vi "SW_Gen_Draw_numbers_and_highllights_DAQmx.vi"(5 "Regions to mark selected":u16[](array[numeric]), 6 "Colors cluster":T2, 7 "Regions to mark set":u16[](array[numeric]), 8 "Input cluster of parameters":T3={"Cage diameter, mm"=8, "Starting angle MIDFIELD"=0, "Starting angle BORDER"=4, "Radius, mm CENTER"=0, "Radius, mm MIDFIELD"=60, "N segments MIDFIELD"=1, "N segments BORDER"=30, "R-gap, mm"=180.0, "Bridge swap"=FALSE, "Bridge H. offset"=0.0, "Bridge V. offset"=0.0, "Twisted neck"=FALSE, "Alt. magn. orientation"=FALSE, "Sensor board size"=enum."Small"} {"Cage diameter, mm" scale=0.0..340.0}, 9 "Image geometrical and scaling parameters":T4, 10 "Bounding rectangles":T5, 11 "Experiment Diagram":T1(plugin-control)) -> (3 "Experiment Diagram out":T1(plugin-control))   [LabVIEW 2018, in "Tracker.lvlib"]
uses:
  Tracker.lvlib
  Controls/CTL_Bounding_Rectangle_of_Segments.ctl
  Controls/CTL_Image_Geometrical_and_scaling_parameters.ctl
  Controls/CTL_Segmented_plot_parameters.ctl
panel:
  in  "Bigger bubble radius":i32=15
  in  "Bubble radius":i16=11
  in  "Font size":i16=18
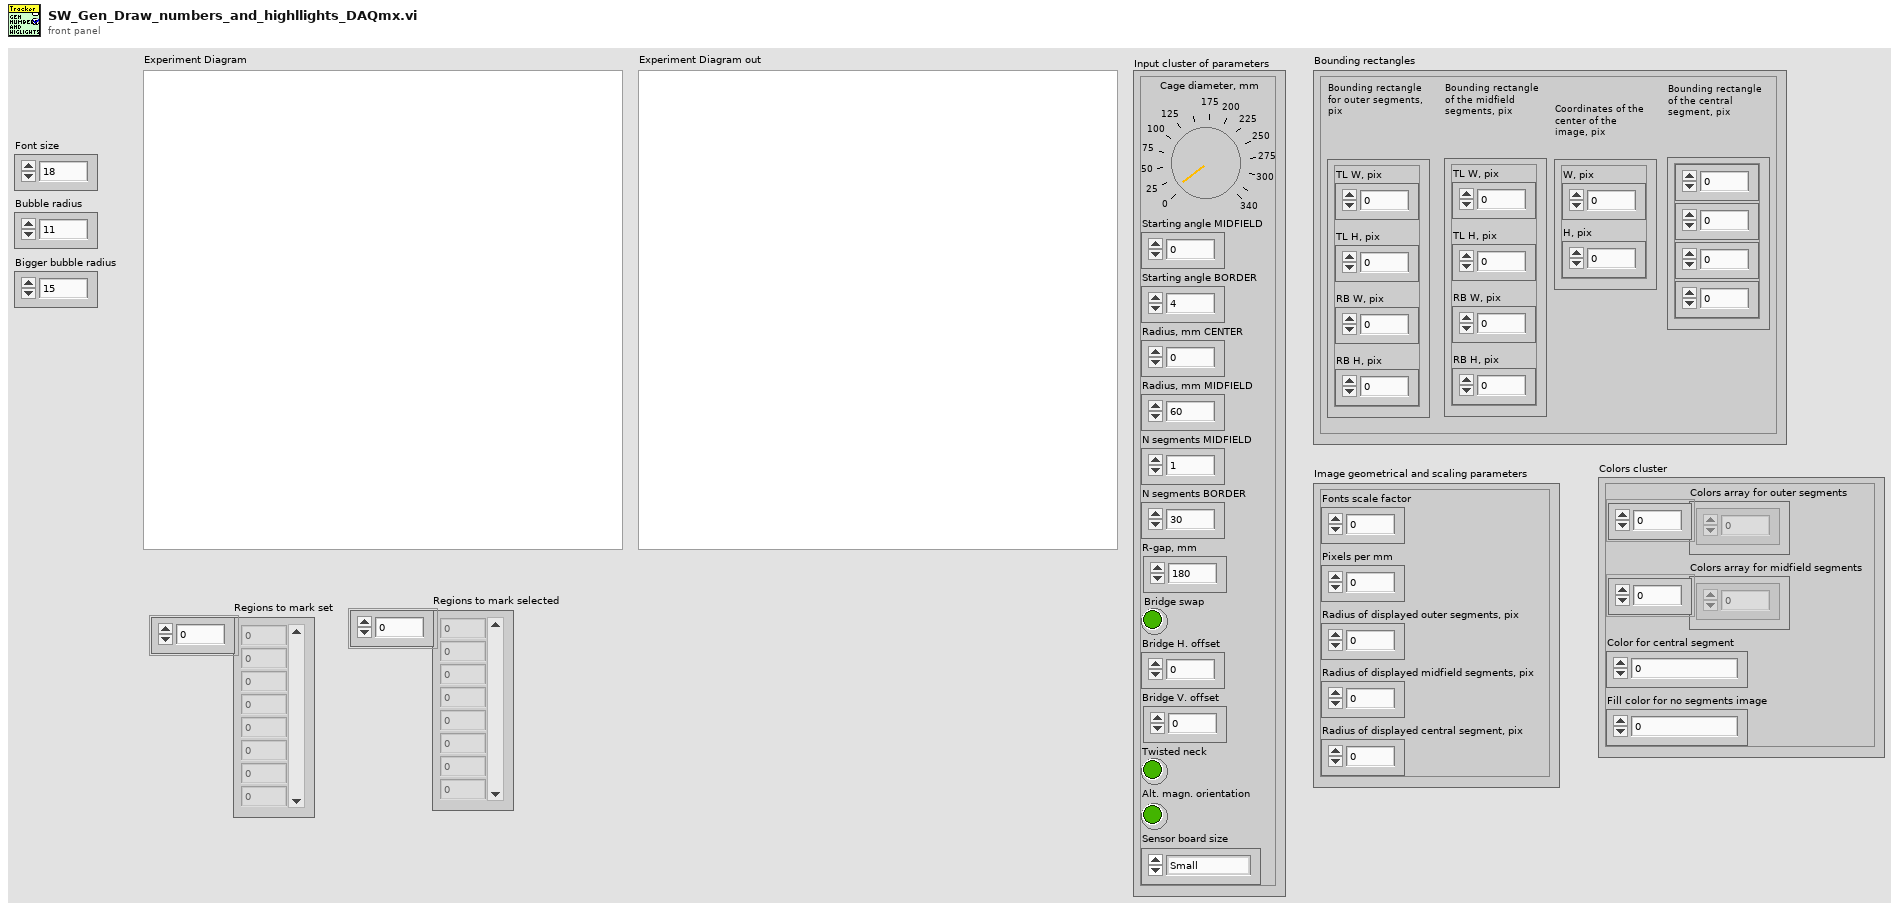
[diagram p1: front panel]
types:
  T1 = typedef "IMAQ Image.ctl" = refnum<image>
  T2 = cluster{"Colors array for outer segments":u32[], "Colors array for midfield segments":u32[], "Color for central segment":u32, "Fill color for no segments image":u32}
  T3 = typedef "Tracker.lvlib/CTL_Segmented_plot_parameters.ctl" = cluster{"Cage diameter, mm":u16, "Starting angle MIDFIELD":i16, "Starting angle BORDER":i16, "Radius, mm CENTER":u16, "Radius, mm MIDFIELD":u16, "N segments MIDFIELD":u8, "N segments BORDER":u8, "R-gap, mm":sgl, "Bridge swap":bool, "Bridge H. offset":sgl, "Bridge V. offset":sgl, "Twisted neck":bool, "Alt. magn. orientation":bool, "Sensor board size":enum16{"Small", "Large"}}
  T4 = typedef "Tracker.lvlib/CTL_Image_Geometrical_and_scaling_parameters.ctl" = cluster{"Fonts scale factor":dbl, "Pixels per mm":dbl, "Radius of displayed outer segments, pix":dbl, "Radius of displayed midfield segments, pix":dbl, "Radius of displayed central segment, pix":dbl}
  T5 = typedef "Tracker.lvlib/CTL_Bounding_Rectangle_of_Segments.ctl" = cluster{"Bounding rectangle for outer segments, pix":cluster{"TL W, pix":i32, "TL H, pix":i32, "RB W, pix":i32, "RB H, pix":i32}, "Bounding rectangle of the midfield segments, pix":cluster{"TL W, pix":i32, "TL H, pix":i32, "RB W, pix":i32, "RB H, pix":i32}, "Coordinates of the center of the image, pix":cluster{"W, pix":i32, "H, pix":i32}, "Bounding rectangle of the central segment, pix":cluster{"Numeric Control":i32, "Numeric Control":i32, "Numeric Control":i32, "Numeric Control":i32}}
  T6 = cluster{"TL W, pix":i32, "TL H, pix":i32, "RB W, pix":i32, "RB H, pix":i32}
  T7 = cluster{"Desired Font (Application)":enum16{"User-specified Font", "Application Font", "System Font", "Dialog Font"}, "[User-specified Font]":cluster{"Font Name":string, "Size":i16, "Strikeout?":bool, "Italic?":bool, "Underline?":bool, "Outline?":bool, "Shadow?":bool, "Bold?":bool, "Rotation Angle":dbl}, "Horizontal Alignment":i16, "Vertical Alignment":i16}
  T8 = cluster{"Top":i32, "Left":i32, "Bottom":i32, "Right":i32}
  T9 = enum16{"User-specified Font", "Application Font", "System Font", "Dialog Font"}
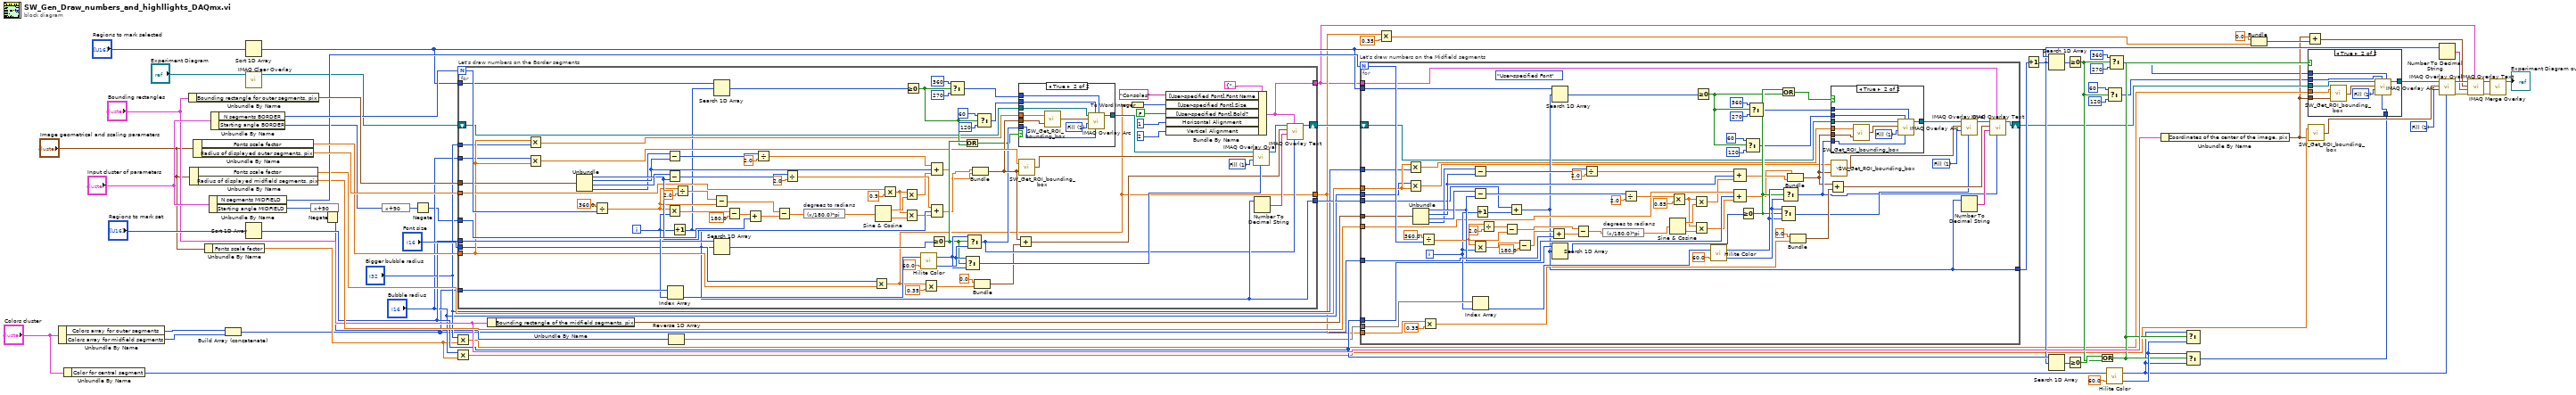
[diagram p0: block diagram]
diagram:
  w27 = u32 1 items=["Frame", "Fill"] ("Drawing Mode (Frame)")
  n1 = Unbundle By Name("Colors cluster") -> ("Colors array for outer segments"=w38:u32[], "Colors array for midfield segments"=w37:u32[])
  n2 = Unbundle By Name("Colors cluster") -> ("Color for central segment"=w52:u32)
  n3 = Unbundle By Name("Bounding rectangles") -> ("Bounding rectangle for outer segments, pix"=w70:T6)
  n4 = Unbundle By Name("Image geometrical and scaling parameters") -> ("Fonts scale factor"=w63:dbl, "Radius of displayed midfield segments, pix"=w62:dbl)
  n5 = Unbundle By Name("Image geometrical and scaling parameters") -> ("Fonts scale factor"=w68:dbl, "Radius of displayed outer segments, pix"=w69:dbl)
  n6 = Unbundle By Name("Image geometrical and scaling parameters") -> ("Fonts scale factor"=w39:dbl)
  n7 = Unbundle By Name("Input cluster of parameters") -> ("N segments MIDFIELD"=w65:u8, "Starting angle MIDFIELD"=w7:i16)
  n8 = Unbundle By Name("Input cluster of parameters") -> ("N segments BORDER"=w67:u8, "Starting angle BORDER"=w8:i16)
  n9 = Build Array (concatenate)(w38, w37) -> (w36:u32[])
  n10 = Sort 1D Array(array="Regions to mark selected") -> (sorted array=w47:u16[])
  n11 = call "IMAQ Clear Overlay"("Image"="Experiment Diagram") -> ("Image Out"=w33:T1)  [unwired: 9 in, 1 out]
  n12 = Sort 1D Array(array="Regions to mark set") -> (sorted array=w51:u16[])
  n13 = expression code="x+90"(w7) -> (w5:i16)
  n14 = Negate(x=w5) -> (-x=w3:i16)
  n15 = expression code="x+90"(w8) -> (w6:i16)
  n16 = Negate(x=w6) -> (-x=w4:i16)
  n17 = Multiply(x="Bigger bubble radius", y=w39) -> (x*y=w30:dbl)
  n18 = Multiply(x="Bubble radius", y=w39) -> (x*y=w19:dbl)
  n19 = for "Let's draw numbers on the Border segments" {
    N: w67 -> [w152]
    tunnel: w4 -> [w153]
    tunnel: w70 -> [w147]
    tunnel: w36 -> [w126]
    tunnel: w69 -> [w123]
    tunnel: w51 -> [w120]
    tunnel: w68 -> [w113]
    tunnel: w47 -> [w112]
    tunnel: "Font size" -> [w106]
    tunnel: "Bubble radius" -> [w105]
    tunnel: "Bigger bubble radius" -> [w104]
    tunnel: [w98] -> w60
    shift-right: [w94] -> w32
    shift-left: w33 -> [w102]
    tunnel: [w79] -> w15
    tunnel: [w78] -> w13
    i -> [w125]
    w97 = u32 1 items=["Frame", "Fill"] ("Drawing Mode (Frame)")
    n20 = Multiply(x=w113, y=w104) -> (x*y=w103:dbl)
    n21 = Multiply(x=w105, y=w113) -> (x*y=w99:dbl)
    n22 = Unbundle(w147) -> ("TL W, pix"=w141:i32, "TL H, pix"=w134:i32, "RB W, pix"=w146:i32, "RB H, pix"=w133:i32)
    n23 = Divide(x=360.0, y=w152) -> (x/y=w127:dbl)
    n24 = Subtract(x=w133, y=w134) -> (x-y=w136:i32)
    n25 = Subtract(x=w146, y=w141) -> (x-y=w144:i32)
    n26 = Multiply(x=w127, y=w125) -> (x*y=w131:dbl)
    n27 = Index Array(array=w126, index=w125) -> (element=w117:u32)
    n28 = Increment(x=w125) -> (x+1=w98:i32)
    n29 = Divide(x=w127, y=2.0) -> (x/y=w129:dbl)
    n30 = Search 1D Array(1D array=w112, element=w98) -> (index of element=w111:i32)  [unwired: 1 in]
    n31 = Subtract(x=w129, y=w127) -> (x-y=w128:dbl)
    n32 = Search 1D Array(1D array=w120, element=w98) -> (index of element=w119:i32)  [unwired: 1 in]
    n33 = Subtract(x=w131, y=180.0) -> (x-y=w132:dbl)
    n34 = Add(x=w132, y=w153) -> (x+y=w150:dbl)
    n35 = Divide(x=w136, y=2.0) -> (x/y=w138:dbl)
    n36 = Subtract(x=w128, y=w150) -> (x-y=w149:dbl)
    n37 = Divide(x=w144, y=2.0) -> (x/y=w142:dbl)
    n38 = expression code="(x/180.0)*pi" "degrees to radians"(w149) -> (w148:dbl)
    n39 = Multiply(x=w106, y=w113) -> (x*y=w79:dbl)
    n40 = Sine & Cosine(0:w148) -> (1:w135:dbl, 2:w145:dbl)
    n41 = Multiply(x=w123, y=0.9) -> (x*y=w122:dbl)
    n42 = Multiply(x=w122, y=w135) -> (x*y=w139:dbl)
    n43 = Multiply(x=w122, y=w145) -> (x*y=w140:dbl)
    n44 = Greater Or Equal To 0?(x=w111) -> (x >= 0?=w108:bool)
    n45 = call <vilib>:"Hilite Color.vi"("Percentage(30)"=60.0, "Color In"=w117) -> ("Shadow"=w116:u32, "Hilite"=w115:u32)
    n46 = Multiply(x=w79, y=0.35) -> (x*y=w84:dbl)
    n47 = Greater Or Equal To 0?(x=w119) -> (x >= 0?=w114:bool)
    n48 = Compound Arithmetic op=ADD(w138, w134, w139) -> (w74:dbl)
    n49 = Compound Arithmetic op=ADD(w142, w141, w140) -> (w75:dbl)
    n50 = Select(t=i16 360, s=w108, f=i16 270 ("arc size(360)")) -> (s? t:f=w76:i16)
    n51 = Or(x=w114, y=w108) -> (x .or. y?=w80:bool)
    n52 = Select(t=w116, s=w114, f=w115) -> (s? t:f=w96:u32)
    n53 = Select(t=w115, s=w114, f=w116) -> (s? t:f=w91:u32)
    n54 = Bundle(w75, w74) -> (w93:cluster{dbl, dbl})  [unwired: 1 in]
    n55 = Bundle(0.0, w84) -> (w81:cluster{dbl, dbl})  [unwired: 1 in]
    n56 = Select(t=i16 60 ("t 2"), s=w108, f=i16 120 ("start angle(0)")) -> (s? t:f=w77:i16)
    n57 = Add(x=w93, y=w81) -> (x+y=w87:cluster{dbl, dbl})
    n58 = case shown="True" w80 {
      tunnel: w93 -> [_ w164]
      tunnel: w103 -> [_ w163]
      tunnel: w102 -> [w155 w161]
      tunnel: w91 -> [_ w160]
      tunnel: [w155 w158] -> w101
      tunnel: w77 -> [_ w157]
      tunnel: w76 -> [_ w156]
      frame False {
      }
      frame True {
        w159 = u32 1 items=["Frame", "Fill"] ("Drawing Mode (Frame)")
        n59 = call "SW_Get_ROI_bounding_box.vi"("Center of the ROI"=w164, "Radius of the ROI, pix"=w163) -> ("Bounding box of the ROI, pix"=w162:T8)
        n60 = call "IMAQ Overlay Arc"("End Angle (degrees)"=w156, "Color"=w160, "Start Angle (degrees)"=w157, "Drawing Mode (Frame)"=w159, "Bounding Rectangle"=w162, "Image"=w161) -> ("Image Out"=w158:T1)  [unwired: 4 in, 1 out]
      }
    }
    n61 = call "SW_Get_ROI_bounding_box.vi"("Center of the ROI"=w93, "Radius of the ROI, pix"=w99) -> ("Bounding box of the ROI, pix"=w100:T8)
    n62 = To Word Integer(number=w79) -> (16bit integer=w73:i16)
    n63 = Bundle By Name(cluster=T7 {"Desired Font (Application)"=enum."System Font", "[User-specified Font]"={"Font Name"="Arial", "Size"=12, "Strikeout?"=FALSE, "Italic?"=FALSE, "Underline?"=FALSE, "Outline?"=FALSE, "Shadow?"=FALSE, "Bold?"=TRUE, "Rotation Angle"=0.0}, "Horizontal Alignment"=1, "Vertical Alignment"=2} ("Font, Size & Style"), "[User-specified Font].Font Name"="Consolas" ("Font Name:"), "[User-specified Font].Size"=w73, "[User-specified Font].Bold?"=FALSE, "Horizontal Alignment"=i16 1, "Vertical Alignment"=i16 2) -> (w78:T7)
    n64 = call "IMAQ Overlay Oval"("Color"=w96, "Drawing Mode (Frame)"=w97, "Bounding Rectangle"=w100, "Image"=w101) -> ("Image Out"=w95:T1)  [unwired: 6 in, 1 out]
    n65 = Number To Decimal String(number=w98) -> (decimal integer string=w92:string)  [unwired: 1 in]
    n66 = call "IMAQ Overlay Text"("Text Color (black)"=w91, "Font, Size & Style"=w78, "String"=w92, "Origin"=w87, "Image"=w95) -> ("Image Out"=w94:T1)  [unwired: 5 in, 1 out]
  }
  n67 = Unbundle By Name("Bounding rectangles") -> ("Bounding rectangle of the midfield segments, pix"=w64:T6)
  n68 = Reverse 1D Array(array=w36) -> (reversed array=w35:u32[])
  n69 = for "Let's draw numbers on the Midfield segments" {
    N: w65 -> [w239]
    tunnel: w3 -> [w240]
    tunnel: w64 -> [w234]
    tunnel: w35 -> [w213]
    tunnel: w62 -> [w210]
    tunnel: w51 -> [w207]
    tunnel: w63 -> [w200]
    tunnel: w47 -> [w198]
    tunnel: "Bubble radius" -> [w192]
    tunnel: "Bigger bubble radius" -> [w191]
    tunnel: w60 -> [w190]
    tunnel: [w189] -> w55
    shift-right: [w171] -> w29
    shift-left: w32 -> [w188]
    tunnel: w15 -> [w178]
    tunnel: w13 -> [w177]
    i -> [w212]
    w185 = u32 1 items=["Frame", "Fill"] ("Drawing Mode (Frame)")
    (unwired) T9."User-specified Font" ("desired font(Application)")
    n70 = Multiply(x=w200, y=w191) -> (x*y=w176:dbl)
    n71 = Multiply(x=w192, y=w200) -> (x*y=w169:dbl)
    n72 = Unbundle(w234) -> ("TL W, pix"=w228:i32, "TL H, pix"=w221:i32, "RB W, pix"=w233:i32, "RB H, pix"=w220:i32)
    n73 = Divide(x=360.0, y=w239) -> (x/y=w214:dbl)
    n74 = Multiply(x=w178, y=0.35) -> (x*y=w182:dbl)
    n75 = Subtract(x=w220, y=w221) -> (x-y=w223:i32)
    n76 = Subtract(x=w233, y=w228) -> (x-y=w231:i32)
    n77 = Multiply(x=w214, y=w212) -> (x*y=w218:dbl)
    n78 = Index Array(array=w213, index=w212) -> (element=w204:u32)
    n79 = Increment(x=w212) -> (x+1=w199:i32)
    n80 = Divide(x=w214, y=2.0) -> (x/y=w216:dbl)
    n81 = Subtract(x=w216, y=w214) -> (x-y=w215:dbl)
    n82 = Add(x=w190, y=w199) -> (x+y=w189:i32)
    n83 = Subtract(x=w218, y=180.0) -> (x-y=w219:dbl)
    n84 = Add(x=w219, y=w240) -> (x+y=w237:dbl)
    n85 = Search 1D Array(1D array=w198, element=w189) -> (index of element=w197:i32)  [unwired: 1 in]
    n86 = Search 1D Array(1D array=w207, element=w189) -> (index of element=w206:i32)  [unwired: 1 in]
    n87 = Subtract(x=w215, y=w237) -> (x-y=w236:dbl)
    n88 = Divide(x=w223, y=2.0) -> (x/y=w225:dbl)
    n89 = expression code="(x/180.0)*pi" "degrees to radians"(w236) -> (w235:dbl)
    n90 = Divide(x=w231, y=2.0) -> (x/y=w229:dbl)
    n91 = Sine & Cosine(0:w235) -> (1:w222:dbl, 2:w232:dbl)
    n92 = Multiply(x=w210, y=0.85) -> (x*y=w209:dbl)
    n93 = Multiply(x=w209, y=w222) -> (x*y=w226:dbl)
    n94 = Multiply(x=w209, y=w232) -> (x*y=w227:dbl)
    n95 = Greater Or Equal To 0?(x=w197) -> (x >= 0?=w194:bool)
    n96 = call <vilib>:"Hilite Color.vi"("Percentage(30)"=60.0, "Color In"=w204) -> ("Shadow"=w203:u32, "Hilite"=w202:u32)
    n97 = Compound Arithmetic op=ADD(w225, w221, w226) -> (w166:dbl)
    n98 = Compound Arithmetic op=ADD(w229, w228, w227) -> (w165:dbl)
    n99 = Greater Or Equal To 0?(x=w206) -> (x >= 0?=w201:bool)
    n100 = Select(t=i16 60 ("t 2"), s=w194, f=i16 120 ("start angle(0)")) -> (s? t:f=w168:i16)
    n101 = Select(t=i16 360, s=w194, f=i16 270 ("arc size(360)")) -> (s? t:f=w167:i16)
    n102 = Select(t=w203, s=w201, f=w202) -> (s? t:f=w174:u32)
    n103 = Or(x=w201, y=w194) -> (x .or. y?=w187:bool)
    n104 = Select(t=w202, s=w201, f=w203) -> (s? t:f=w172:u32)
    n105 = Bundle(w165, w166) -> (w170:cluster{dbl, dbl})  [unwired: 1 in]
    n106 = Bundle(0.0, w182) -> (w179:cluster{dbl, dbl})  [unwired: 1 in]
    n107 = Add(x=w170, y=w179) -> (x+y=w183:cluster{dbl, dbl})
    n108 = case shown="True" w187 {
      tunnel: w170 -> [_ w251]
      tunnel: w176 -> [_ w250]
      tunnel: w188 -> [w242 w248]
      tunnel: w172 -> [_ w247]
      tunnel: [w242 w245] -> w175
      tunnel: w168 -> [_ w244]
      tunnel: w167 -> [_ w243]
      frame False {
      }
      frame True {
        w246 = u32 1 items=["Frame", "Fill"] ("Drawing Mode (Frame)")
        n109 = call "SW_Get_ROI_bounding_box.vi"("Center of the ROI"=w251, "Radius of the ROI, pix"=w250) -> ("Bounding box of the ROI, pix"=w249:T8)
        n110 = call "IMAQ Overlay Arc"("End Angle (degrees)"=w243, "Color"=w247, "Start Angle (degrees)"=w244, "Drawing Mode (Frame)"=w246, "Bounding Rectangle"=w249, "Image"=w248) -> ("Image Out"=w245:T1)  [unwired: 4 in, 1 out]
      }
    }
    n111 = call "SW_Get_ROI_bounding_box.vi"("Center of the ROI"=w170, "Radius of the ROI, pix"=w169) -> ("Bounding box of the ROI, pix"=w186:T8)
    n112 = call "IMAQ Overlay Oval"("Color"=w174, "Drawing Mode (Frame)"=w185, "Bounding Rectangle"=w186, "Image"=w175) -> ("Image Out"=w184:T1)  [unwired: 6 in, 1 out]
    n113 = Number To Decimal String(number=w189) -> (decimal integer string=w173:string)  [unwired: 1 in]
    n114 = call "IMAQ Overlay Text"("Text Color (black)"=w172, "Font, Size & Style"=w177, "String"=w173, "Origin"=w183, "Image"=w184) -> ("Image Out"=w171:T1)  [unwired: 5 in, 1 out]
  }
  n115 = Multiply(x=w15, y=0.35) -> (x*y=w24:dbl)
  n116 = Increment(x=w55) -> (x+1=w46:i32)
  n117 = Search 1D Array(1D array=w47, element=w46) -> (index of element=w48:i32)  [unwired: 1 in]
  n118 = Search 1D Array(1D array=w51, element=w46) -> (index of element=w57:i32)  [unwired: 1 in]
  n119 = Greater Or Equal To 0?(x=w48) -> (x >= 0?=w41:bool)
  n120 = Greater Or Equal To 0?(x=w57) -> (x >= 0?=w59:bool)
  n121 = Or(x=w59, y=w41) -> (x .or. y?=w31:bool)
  n122 = Select(t=i16 60 ("t 2"), s=w41, f=i16 120 ("start angle(0)")) -> (s? t:f=w17:i16)
  n123 = call <vilib>:"Hilite Color.vi"("Percentage(30)"=60.0, "Color In"=w52) -> ("Shadow"=w58:u32, "Hilite"=w1:u32)
  n124 = Select(t=i16 360, s=w41, f=i16 270 ("arc size(360)")) -> (s? t:f=w16:i16)
  n125 = Unbundle By Name("Bounding rectangles") -> ("Coordinates of the center of the image, pix"=w18:cluster{"W, pix":i32, "H, pix":i32})
  n126 = Select(t=w1, s=w31, f=w58) -> ()  [unwired: 1 out]
  n127 = Select(t=w58, s=w31, f=w1) -> (s? t:f=w2:u32)
  n128 = Bundle(0.0, w24) -> (w21:cluster{dbl, dbl})  [unwired: 1 in]
  n129 = Add(x=w18, y=w21) -> (x+y=w25:cluster{dbl, dbl})
  n130 = case shown="True" w31 {
    tunnel: w18 -> [_ w261]
    tunnel: w30 -> [_ w260]
    tunnel: w29 -> [w252 w258]
    tunnel: [w252 w256] -> w20
    tunnel: w17 -> [_ w255]
    tunnel: w16 -> [_ w254]
    tunnel: w2 -> [_ w253]
    frame False {
    }
    frame True {
      w257 = u32 1 items=["Frame", "Fill"] ("Drawing Mode (Frame)")
      n131 = call "SW_Get_ROI_bounding_box.vi"("Center of the ROI"=w261, "Radius of the ROI, pix"=w260) -> ("Bounding box of the ROI, pix"=w259:T8)
      n132 = call "IMAQ Overlay Arc"("End Angle (degrees)"=w254, "Color"=w253, "Start Angle (degrees)"=w255, "Drawing Mode (Frame)"=w257, "Bounding Rectangle"=w259, "Image"=w258) -> ("Image Out"=w256:T1)  [unwired: 4 in, 1 out]
    }
  }
  n133 = call "SW_Get_ROI_bounding_box.vi"("Center of the ROI"=w18, "Radius of the ROI, pix"=w19) -> ("Bounding box of the ROI, pix"=w28:T8)
  n134 = Number To Decimal String(number=w46) -> (decimal integer string=w14:string)  [unwired: 1 in]
  n135 = call "IMAQ Overlay Oval"("Color"=w1, "Drawing Mode (Frame)"=w27, "Bounding Rectangle"=w28, "Image"=w20) -> ("error out"=w10:errorcluster, "Image Out"=w26:T1)  [unwired: 6 in]
  n136 = call "IMAQ Overlay Text"("Font, Size & Style"=w13, "error in (no error)"=w10, "String"=w14, "Origin"=w25, "Image"=w26) -> ("error out"=w9:errorcluster, "Image Out"=w11:T1)  [unwired: 5 in]
  n137 = call "IMAQ Merge Overlay"("error in (no error)"=w9, "Image Src"=w11) -> ("Image Dst Out"=→"Experiment Diagram out":T1)  [unwired: 8 in, 1 out]
